vi "simple Shift string array.vi"(10 "Element in":string, 11 "Array in":string[](array[string])) -> (2 "Element out":string, 3 "Array out":string[](array[string]))   [LabVIEW 2021, in "MatS Libs.lvlib"]
doc: "Inserts a new string and pops out the last one. Useful for circular buffer of strings or logger of limitted text messages."
uses:
  <userlib>/MatS Libs/MatS Libs.lvlib
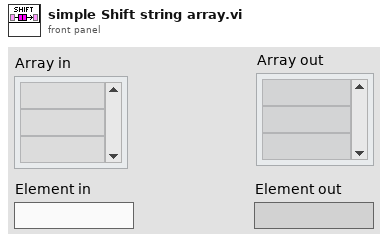
[diagram p1: front panel]
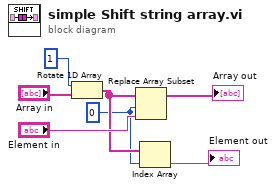
[diagram p0: block diagram]
diagram:
  w2 = 0 ("index")
  n1 = Rotate 1D Array(1:"Array in", 2:1 ("n")) -> (0:w3:string[])
  n2 = Replace Array Subset(array=w3, new element="Element in", index=w2) -> (→"Array out":string[])
  n3 = Index Array(array=w3, index=w2) -> (element=→"Element out":string)
